vi "TemperatureDAQExample_sub.vi"(1 "stop flag":bool, 2 "tdms file":refnum<k34>, 3 "error in (no error)":errorcluster) -> (7 "error out":errorcluster)   [LabVIEW 2024]
uses:
  <vilib>/Analysis/baseanly.llb/Mean (DBL).vi
  <vilib>/DAQmx/create/channels.llb/DAQmx Create Channel (AI-Temperature-Thermocouple).vi
  <vilib>/DAQmx/configure/trigger.llb/DAQmx Start Trigger (Digital Edge).vi
  <vilib>/Analysis/NI_AALBase.lvlib
panel:
  out "file path out":path
  out "mean 2":dbl format="%0.2f"
  out "mean 3":dbl format="%0.2f"
  out "mean 4":dbl format="%0.2f"
  out "mean 5":dbl format="%0.2f"
  out "data 5":dynamicdata(graph) caption="data"
  out "data 4":dynamicdata(graph) caption="data"
  out "mean 0":dbl format="%0.2f"
  out "data 3":dynamicdata(graph) caption="data"
  out "data 2":dynamicdata(graph) caption="data"
  out "data 1":dynamicdata(graph) caption="data"
  out "data 0":dynamicdata(graph) caption="data"
  out "mean 1":dbl format="%0.2f"
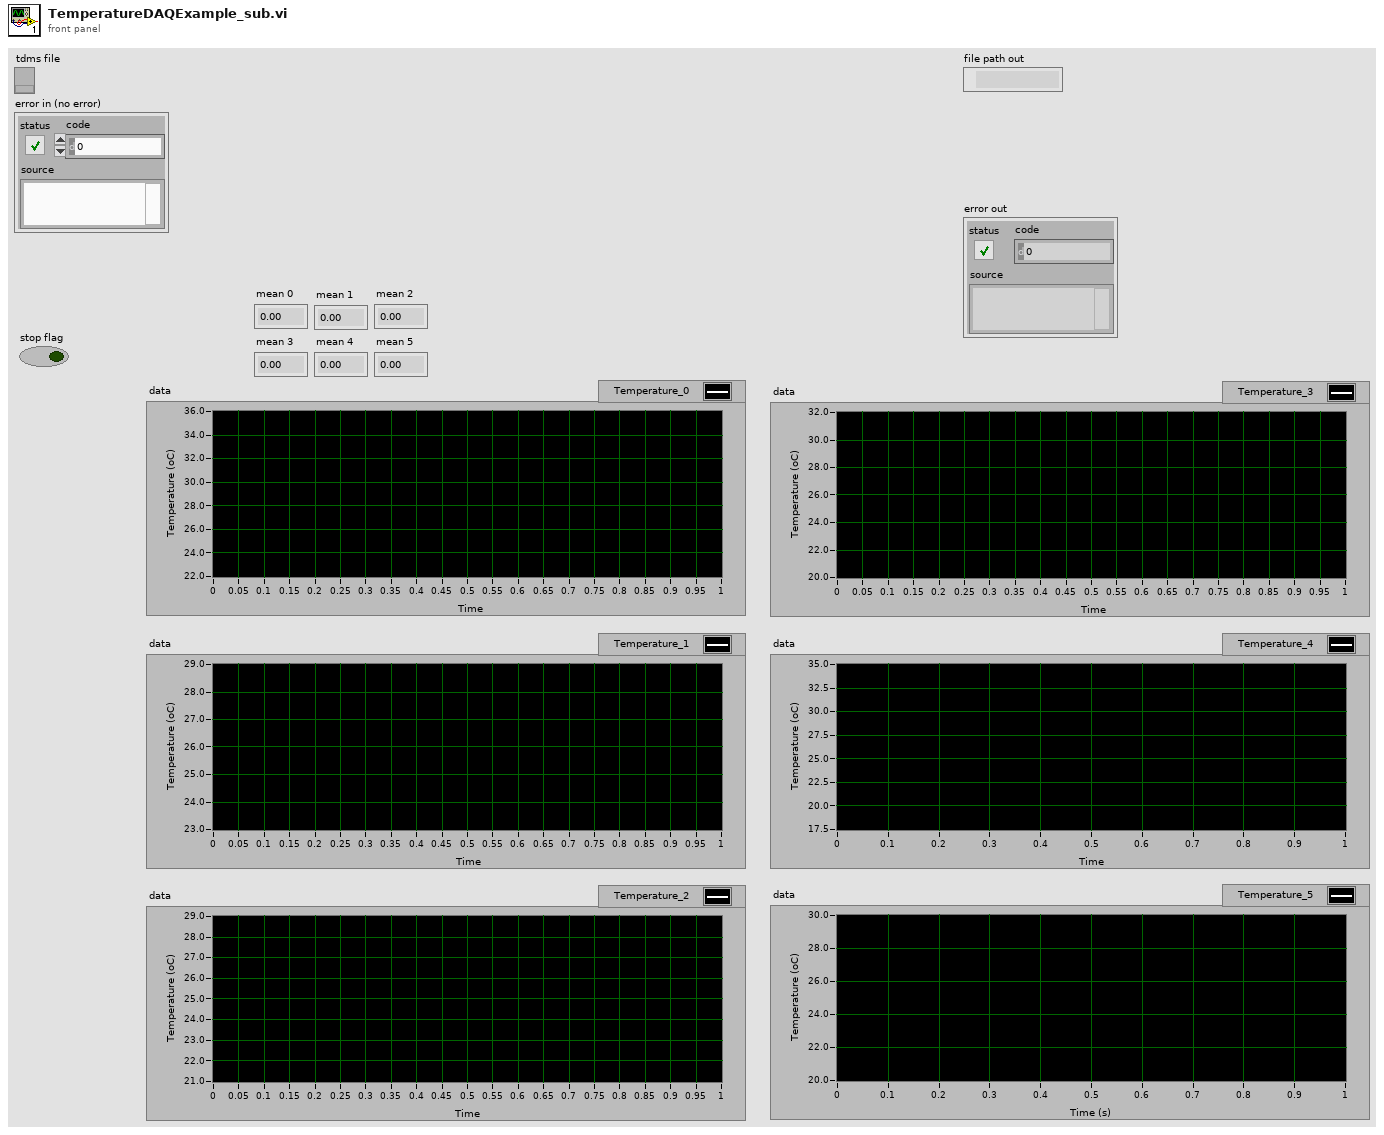
[diagram p1: front panel]
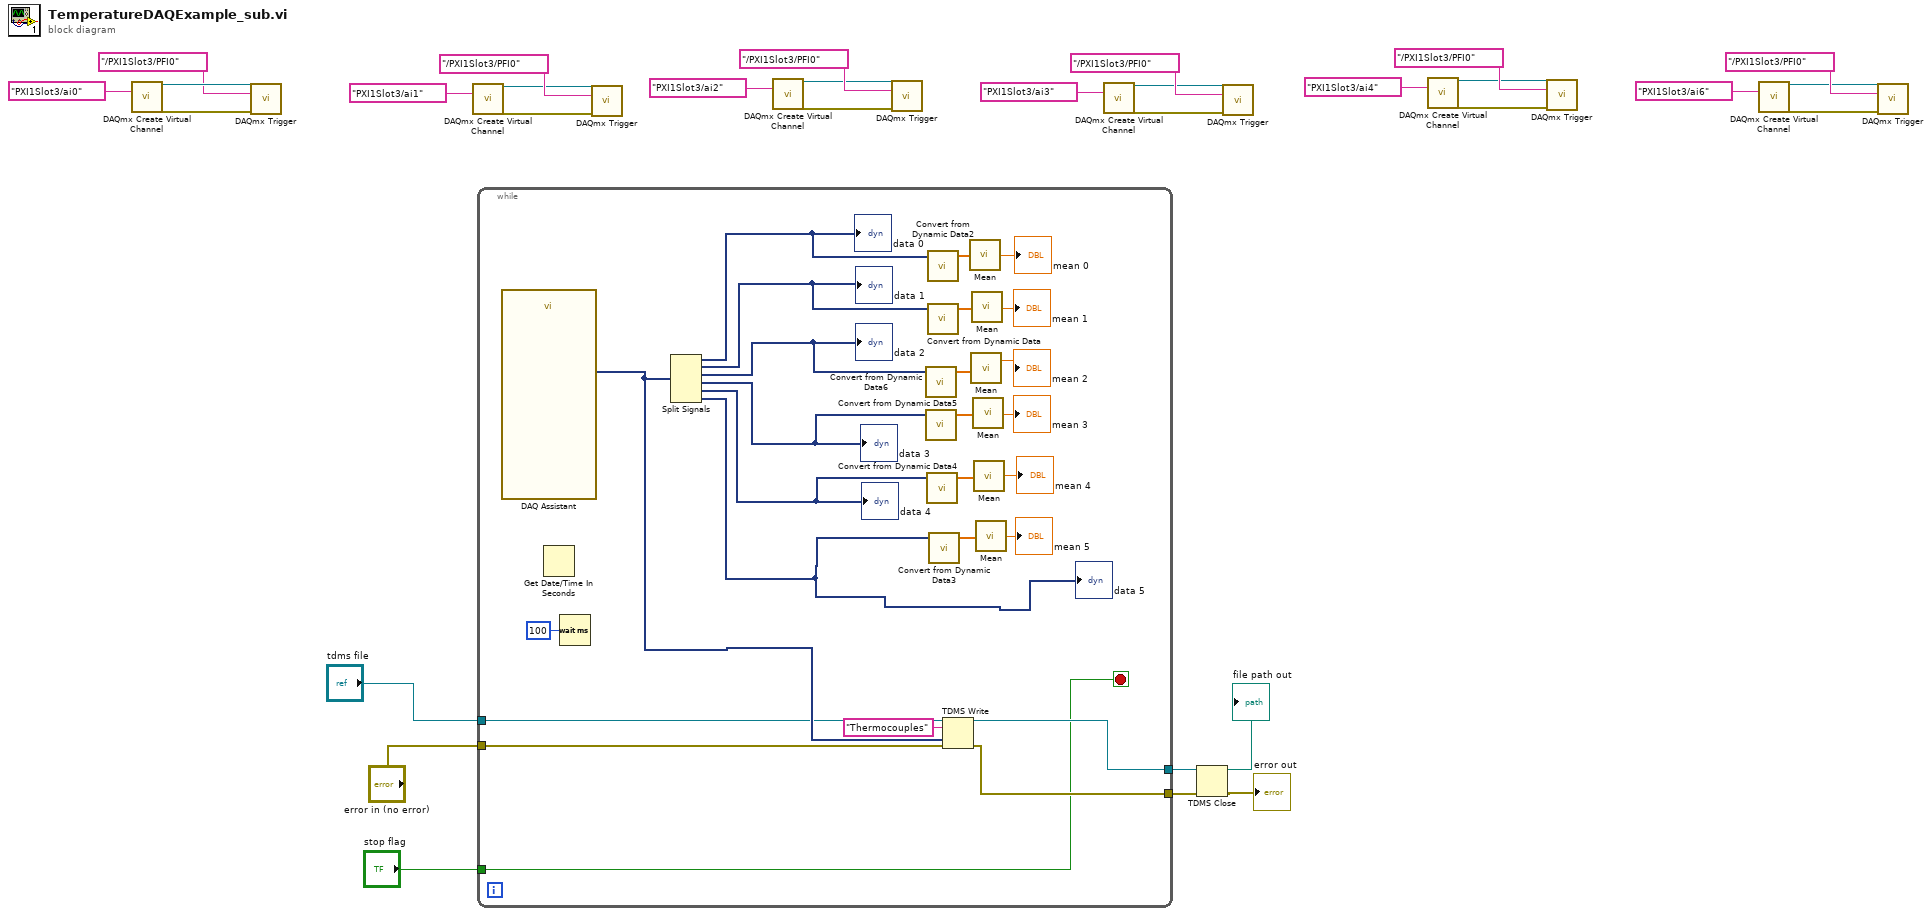
[diagram p0: block diagram]
diagram:
  n1 = call-poly <vilib>:"DAQmx Create Virtual Channel.vi"("physical channels"=tag "PXI1Slot3/ai0") -> ("task out"=w30:refnum<k21>, "error out"=w29:errorcluster)  [unwired: 13 in]
  n2 = call-poly <vilib>:"DAQmx Trigger.vi"("task/channels in"=w30, "source"=tag "/PXI1Slot3/PFI0", "error in"=w29) -> ()  [unwired: 11 in, 2 out]
  n3 = call-poly <vilib>:"DAQmx Create Virtual Channel.vi"("physical channels"=tag "PXI1Slot3/ai1") -> ("task out"=w24:refnum<k21>, "error out"=w26:errorcluster)  [unwired: 13 in]
  n4 = while {
    tunnel: [w54] -> w23
    tunnel: [w53] -> w22
    tunnel: "tdms file" -> [w34]
    tunnel: "error in (no error)" -> [w33]
    tunnel: "stop flag" -> [w32]
    stop <- w32 stop-if-true
    n5 = call "DAQ Assistant"() -> ("data"=w37:dynamicdata)  [unwired: 17 in, 2 out]
    n6 = Get Date/Time In Seconds() -> ()  [unwired: 1 out]
    n7 = Wait (ms)(milliseconds to wait=u32 100) -> ()  [unwired: 1 out]
    n8 = Split Signals(w37) -> (w49:dynamicdata, w55:dynamicdata, w40:dynamicdata, w39:dynamicdata, w38:dynamicdata, w36:dynamicdata)  [unwired: 6 in]
    "data 0" <- w49
    "data 1" <- w55
    "data 2" <- w40
    "data 3" <- w39
    "data 4" <- w38
    "data 5" <- w36
    n9 = call "Convert from Dynamic Data6"("Dynamic Data Type"=w40) -> ("Array"=w42:dbl[])  [unwired: 3 in]
    n10 = call "Convert from Dynamic Data5"("Dynamic Data Type"=w39) -> ("Array"=w44:dbl[])  [unwired: 3 in]
    n11 = call "Convert from Dynamic Data4"("Dynamic Data Type"=w38) -> ("Array"=w46:dbl[])  [unwired: 3 in]
    n12 = call "Convert from Dynamic Data2"("Dynamic Data Type"=w49) -> ("Array"=w51:dbl[])  [unwired: 3 in]
    n13 = call "Convert from Dynamic Data"("Dynamic Data Type"=w55) -> ("Array"=w57:dbl[])  [unwired: 3 in]
    n14 = call "Convert from Dynamic Data3"("Dynamic Data Type"=w36) -> ("Array"=w48:dbl[])  [unwired: 3 in]
    n15 = TDMS Write(0:w34, 5:"Thermocouples" ("group name in (Untitled)"), 9:w37, 11:w33) -> (4:w53:refnum<k34>, 15:w54:errorcluster)  [unwired: 2 in, 2 out]
    n16 = call-poly <vilib>:"Mean.vi"("X"=w51) -> ("mean"=→"mean 0":dbl)  [unwired: 1 out]
    n17 = call-poly <vilib>:"Mean.vi"("X"=w42) -> ("mean"=→"mean 2":dbl)  [unwired: 1 out]
    n18 = call-poly <vilib>:"Mean.vi"("X"=w57) -> ("mean"=→"mean 1":dbl)  [unwired: 1 out]
    n19 = call-poly <vilib>:"Mean.vi"("X"=w44) -> ("mean"=→"mean 3":dbl)  [unwired: 1 out]
    n20 = call-poly <vilib>:"Mean.vi"("X"=w46) -> ("mean"=→"mean 4":dbl)  [unwired: 1 out]
    n21 = call-poly <vilib>:"Mean.vi"("X"=w48) -> ("mean"=→"mean 5":dbl)  [unwired: 1 out]
  }
  n22 = call-poly <vilib>:"DAQmx Trigger.vi"("task/channels in"=w24, "source"=tag "/PXI1Slot3/PFI0", "error in"=w26) -> ()  [unwired: 11 in, 2 out]
  n23 = call-poly <vilib>:"DAQmx Create Virtual Channel.vi"("physical channels"=tag "PXI1Slot3/ai2") -> ("task out"=w18:refnum<k21>, "error out"=w20:errorcluster)  [unwired: 13 in]
  n24 = call-poly <vilib>:"DAQmx Trigger.vi"("task/channels in"=w18, "source"=tag "/PXI1Slot3/PFI0", "error in"=w20) -> ()  [unwired: 11 in, 2 out]
  n25 = call-poly <vilib>:"DAQmx Create Virtual Channel.vi"("physical channels"=tag "PXI1Slot3/ai3") -> ("task out"=w14:refnum<k21>, "error out"=w16:errorcluster)  [unwired: 13 in]
  n26 = TDMS Close(8:w23, 11:w22) -> (0:→"error out":errorcluster, 3:→"file path out":path)
  n27 = call-poly <vilib>:"DAQmx Trigger.vi"("task/channels in"=w14, "source"=tag "/PXI1Slot3/PFI0", "error in"=w16) -> ()  [unwired: 11 in, 2 out]
  n28 = call-poly <vilib>:"DAQmx Create Virtual Channel.vi"("physical channels"=tag "PXI1Slot3/ai4") -> ("task out"=w10:refnum<k21>, "error out"=w12:errorcluster)  [unwired: 13 in]
  n29 = call-poly <vilib>:"DAQmx Trigger.vi"("task/channels in"=w10, "source"=tag "/PXI1Slot3/PFI0", "error in"=w12) -> ()  [unwired: 11 in, 2 out]
  n30 = call-poly <vilib>:"DAQmx Create Virtual Channel.vi"("physical channels"=tag "PXI1Slot3/ai6") -> ("task out"=w6:refnum<k21>, "error out"=w8:errorcluster)  [unwired: 13 in]
  n31 = call-poly <vilib>:"DAQmx Trigger.vi"("task/channels in"=w6, "source"=tag "/PXI1Slot3/PFI0", "error in"=w8) -> ()  [unwired: 11 in, 2 out]
